vi "Debug - TCP - Create Descriptive String.vi"(9 "Data Received":string, 10 "Data Written":string, 11 "TCP Network Connection in":refnum<k5>) -> (2 "Transmission Log":string)   [LabVIEW 2017, in "Communications Library.lvlib"]
doc: "Creates a string describing the TCP communication which has occured."
uses:
  Communications Library.lvlib
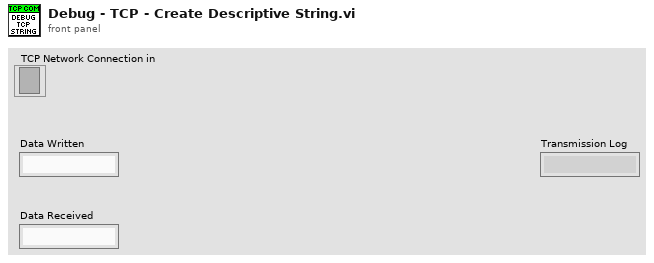
[diagram p1: front panel]
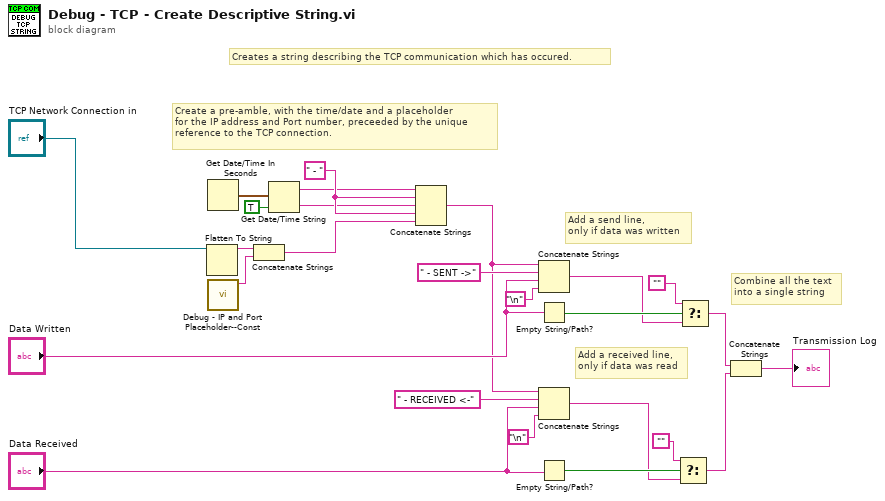
[diagram p0: block diagram]
diagram:
  w25 = " - " ("string")
  # "Combine all the text\ninto a single string"
  # "Add a received line, \nonly if data was read"
  # "Add a send line, \nonly if data was written"
  # "Create a pre-amble, with the time/date and a placeholder\nfor the IP address and Port number, preceeded by the unique\nreference to the TCP connection."
  # "Creates a string describing the TCP communication which has occured."
  n1 = Flatten To String(anything="TCP Network Connection in") -> (data string=w21:string)  [unwired: 3 in, 2 out]
  n2 = Get Date/Time In Seconds() -> (seconds since 1Jan1904=w19:timestamp)
  n3 = call "Debug - IP and Port Placeholder--Const.vi"() -> ("Debug Placeholder"=w22:string)  [unwired: 11 in]
  n4 = Concatenate Strings(w21, w22) -> (w13:string)
  n5 = Get Date/Time String(seconds (now)=w19, want seconds? (F)=TRUE) -> (date string=w24:string, time string=w23:string)  [unwired: 1 in]
  n6 = Concatenate Strings(w24, w25, w23, w25, w13) -> (w1:string)
  n7 = Concatenate Strings(w1, " - SENT ->", "Data Written", "\n") -> (w7:string)
  n8 = Empty String/Path?(string/path="Data Written") -> (empty?=w17:bool)
  n9 = Concatenate Strings(w1, " - RECEIVED <-", "Data Received", "\n") -> (w10:string)
  n10 = Empty String/Path?(string/path="Data Received") -> (empty?=w15:bool)
  n11 = Select(t="", s=w15, f=w10) -> (s? t:f=w4:string)
  n12 = Select(t="", s=w17, f=w7) -> (s? t:f=w6:string)
  n13 = Concatenate Strings(w6, w4) -> (→"Transmission Log":string)
